vi "Get Buffer (ms).vi"(3 "Buffer (size)":u32, 5 "Buffer (units)":string(combo)="Minutes") -> (1 "Buffer (ms)":u32)   [LabVIEW 2009]
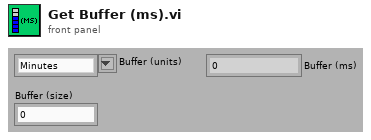
[diagram p1: front panel]
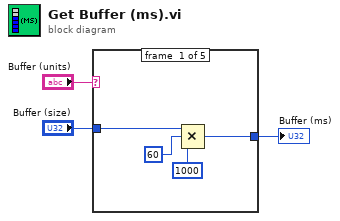
[diagram p0: block diagram]
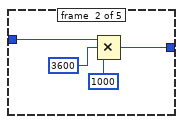
[diagram p2: hidden frame]
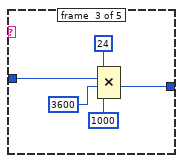
[diagram p3: hidden frame]
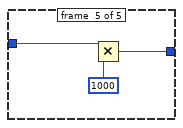
[diagram p5: hidden frame]
diagram:
  n1 = case shown="\"Days\"" "Buffer (units)" {
    tunnel: "Buffer (size)" -> [w5 w9 w14 w17 w19]
    tunnel: [w4 w8 w12 w17 w18] -> w1
    frame #0 {
      n2 = Compound Arithmetic op=MULTIPLY(w5, u32 60 ("y"), u32 1000 ("value")) -> (w4:u32)
    }
    frame #1 {
      n3 = Compound Arithmetic op=MULTIPLY(w9, u32 3600 ("y"), u32 1000 ("value")) -> (w8:u32)
    }
    frame #2 {
      n4 = Compound Arithmetic op=MULTIPLY(u32 24 ("value"), w14, u32 3600 ("y"), u32 1000 ("value")) -> (w12:u32)
    }
    frame #3 {
    }
    frame #4 {
      n5 = Multiply(x=w19, y=u32 1000 ("value")) -> (x*y=w18:u32)
    }
  }
  "Buffer (ms)" <- w1
